vi "Autosize Table Columns rev1.vi"(4 "error in (no error)":errorcluster, 6 "Resize Table?":bool, 7 "Table Ref":refnum<vi>) -> (0 "error out":errorcluster)   [LabVIEW 2015]
doc: "This VI resizes each column of the table specified by Table Ref based on the widest entry of the column. Additionally, if Resize Table? is TRUE, the VI will set the table width based on the number of populated columns."
panel:
  # "This was found in NI Discussion Forum named as Autosize Table Columns.vi, by ceger\nhttp://forums.ni.com/ni/board/message?board.id=170&message.id=356189"
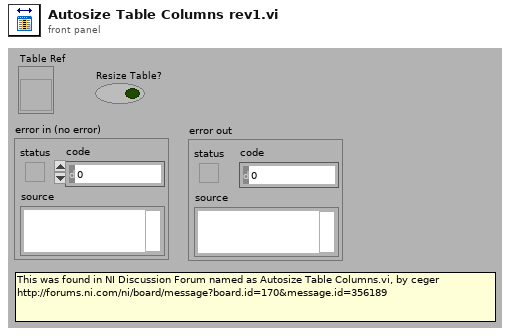
[diagram p1: front panel]
types:
  T1 = enum16{"User-specified Font", "Application Font", "System Font", "Dialog Font"}
  T2 = cluster{"Font Name:":string, "Size":i16, "Strikeout?":bool, "Italic?":bool, "Underline?":bool, "Outline?":bool, "Shadow?":bool, "Bold?":bool}
  T3 = cluster{"left":i16, "top":i16, "right":i16, "bottom":i16}
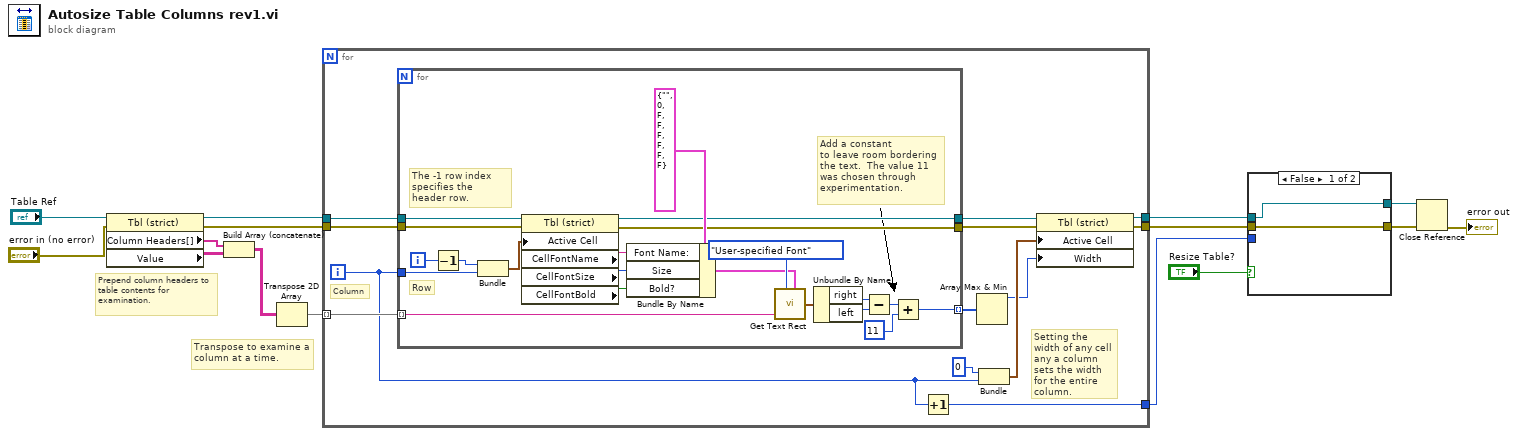
[diagram p0: block diagram]
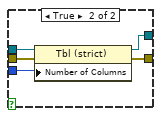
[diagram p2: hidden frame]
diagram:
  # "Transpose to examine a column at a time."
  # "Prepend column headers to table contents for examination."
  n1 = property class="Tbl (strict)"(reference="Table Ref", error in="error in (no error)") -> (reference out=w15:refnum<vi>, error out=w11:errorcluster, "Column Headers[]"=w14:string[], "Value"=w10:string[][])
  n2 = Build Array (concatenate)(w14, w10) -> (w13:string[][])
  n3 = Transpose 2D Array(2D array=w13) -> (transposed array=w12:string[][])
  n4 = for {
    tunnel: w12 -> [w28] mode=indexing
    tunnel: w15 -> [w27]
    tunnel: w11 -> [w25]
    tunnel: [w19] -> w5
    tunnel: [w18] -> w6
    tunnel: [w16] -> w4
    i -> [w17]
    # "Setting the width of any cell any a column sets the width for the entire column."
    # "Column"
    n5 = for {
      tunnel: w28 -> [w41] mode=indexing
      tunnel: w27 -> [w49]
      tunnel: w17 -> [w48]
      tunnel: [w30] -> w26 mode=indexing
      tunnel: w25 -> [w35]
      tunnel: [w34] -> w23
      tunnel: [w33] -> w24
      i -> [w37]
      # "The -1 row index specifies the header row."
      # "Add a constant\nto leave room bordering the text.  The value 11 was chosen through experimentation."
      # "Row"
      n6 = Decrement(x=w37) -> (x-1=w36:i32)
      n7 = Bundle(w36, w48) -> (w47:cluster{i32, i32})  [unwired: 1 out]
      n8 = property class="Tbl (strict)"(reference=w49, error in=w35, "Active Cell"=w47) -> (reference out=w33:refnum<vi>, error out=w34:errorcluster, "CellFontName"=w45:string, "CellFontSize"=w31:u32, "CellFontBold"=w44:bool)
      n9 = Bundle By Name(cluster=T2 {"Font Name:"="", "Size"=0, "Strikeout?"=FALSE, "Italic?"=FALSE, "Underline?"=FALSE, "Outline?"=FALSE, "Shadow?"=FALSE, "Bold?"=FALSE} ("[user-specified font]"), "Font Name:"=w45, "Size"=w31, "Bold?"=w44) -> (w42:T2)
      n10 = call <vilib>:"Get Text Rect.vi"("desired font(Application)"=T1."User-specified Font", "text"=w41, "[user-specified font]"=w42) -> ("rect"=w40:T3)  [unwired: 3 in, 3 out]
      n11 = Unbundle By Name(w40) -> ("right"=w39:i16, "left"=w38:i16)
      n12 = Subtract(x=w39, y=w38) -> (x-y=w32:i16)
      n13 = Add(x=w32, y=i16 11) -> (x+y=w30:i16)
    }
    n14 = Increment(x=w17) -> (x+1=w16:i32)
    n15 = Array Max & Min(array=w26) -> (max value=w20:i16)  [unwired: 3 out]
    n16 = Bundle(0, w17) -> (w21:cluster{i32, i32})  [unwired: 1 out]
    n17 = property class="Tbl (strict)"(reference=w24, error in=w23, "Active Cell"=w21, "Width"=w20) -> (reference out=w18:refnum<vi>, error out=w19:errorcluster)
  }
  n18 = case shown="False" "Resize Table?" {
    tunnel: w6 -> [w50 w56]
    tunnel: w5 -> [w51 w55]
    tunnel: w4 -> [_ w54]
    tunnel: [w51 w53] -> w3
    tunnel: [w50 w52] -> w2
    frame False {
    }
    frame True {
      n19 = property class="Tbl (strict)"(reference=w56, error in=w55, "Number of Columns"=w54) -> (reference out=w52:refnum<vi>, error out=w53:errorcluster)
    }
  }
  n20 = Close Reference(reference=w2, error in (no error)=w3) -> (error out=→"error out":errorcluster)
